vi "TDC_getHbtFitStartParams.vi"(8 "Error In":errorcluster, 11 "Fit Type":u16(ring) items=["None", "Coherent", "Thermal", "Single", "Antibunch", "Thermal+Jitter", "Single+Jitter", "Antibunch+Jitter", "Thermal+Offset", "Single+Offset", "Antibunch+Offset", "Thermal+Jitter+Offs", "Single+Jitter+Offs", "Antibunch+Jitter+Offs"]) -> (0 "Error Out":errorcluster, 3 "Fit Parameters":dbl[](array[numeric]))   [LabVIEW 2011]
uses:
  tdcbase.dll
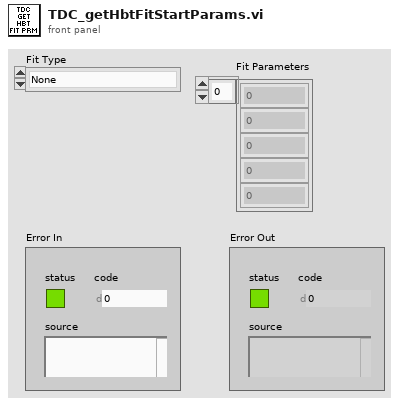
[diagram p1: front panel]
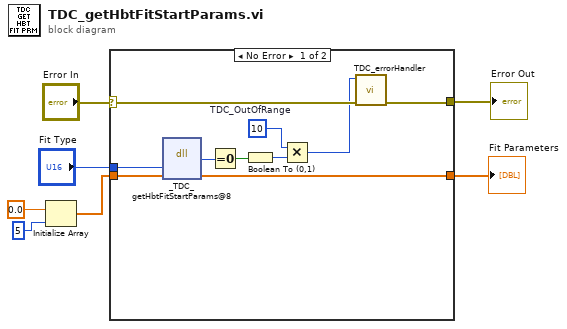
[diagram p0: block diagram]
diagram:
  n1 = Initialize Array(0.0, 5) -> (w2:dbl[])
  n2 = case shown="No Error" "Error In" {
    selector: "Error In" -> [w17 w19]
    tunnel: [w16 w19] -> w6
    tunnel: "Fit Type" -> [w13 _]
    tunnel: w2 -> [w15 w18]
    tunnel: [w14 w18] -> w1
    frame No Error {
      w8 = 10  # TDC_OutOfRange
      n3 = dll-call lib="X:/tdcbase.dll" fn="_TDC_getHbtFitStartParams@8"("fct"=w13, "fitParams"=w15) -> ("return type"=w12:u64, "fitParams"=w14:dbl[])  [unwired: 4 in, 2 out]
      n4 = Equal To 0?(x=w12) -> (x = 0?=w11:bool)
      n5 = Boolean To (0,1)(Boolean=w11) -> (0, 1=w10:i16)
      n6 = Multiply(x=w8, y=w10) -> (x*y=w9:i32)
      n7 = call "TDC_errorHandler.vi"("Error In"=w17, "TDC Return Code"=w9) -> ("Error Out"=w16:errorcluster)  [unwired: 9 in]
    }
    frame Error {
    }
  }
  "Error Out" <- w6
  "Fit Parameters" <- w1
